vi "ni579x Amplitude Data Interpolator.vi"(8 "Error In":errorcluster, 9 "attenuation index":dbl, 10 "frequency [Hz]":dbl format="%#_6p", 11 "characterization data":T1 {"Frequencies [Hz]" format="%#_6p"}) -> (0 "Error Out":errorcluster, 1 "attenuator values [dB]":dbl[](array[numeric]), 2 "amplitude data":dbl)   [LabVIEW 2013]
uses:
  <instrlib>/ni579x/Config/v1/Shared/Types/ni579x Characterization Data.ctl
  <instrlib>/ni579x/Config/v1/Shared/Types/ni579x IQ Imbalance.ctl
  <instrlib>/ni579x/Config/v1/Shared/Types/ni579x Gain to Attenuation Mapping.ctl
  <vilib>/gmath/interp.llb/Interpolate 2D (1d xi,yi).vi
  <vilib>/gmath/NI_Gmath.lvlib
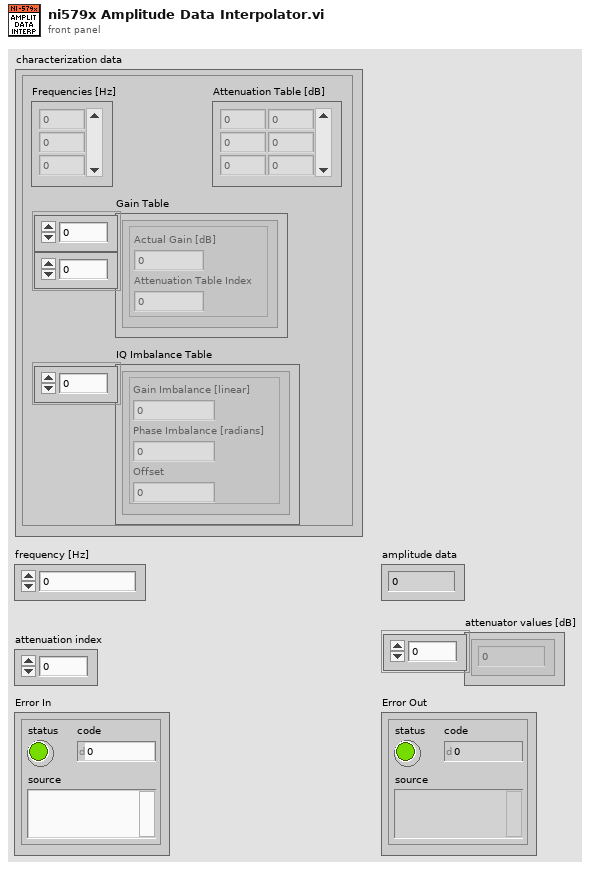
[diagram p1: front panel]
types:
  T1 = typedef "ni579x Characterization Data.ctl" = cluster{"Attenuation Table [dB]":dbl[][], "Frequencies [Hz]":dbl[], "IQ Imbalance Table":T2[], "Gain Table":T3[][]}
  T2 = typedef "ni579x IQ Imbalance.ctl" = cluster{"Gain Imbalance [linear]":dbl, "Phase Imbalance [radians]":dbl, "Offset":cdb}
  T3 = typedef "ni579x Gain to Attenuation Mapping.ctl" = cluster{"Actual Gain [dB]":dbl, "Attenuation Table Index":i32}
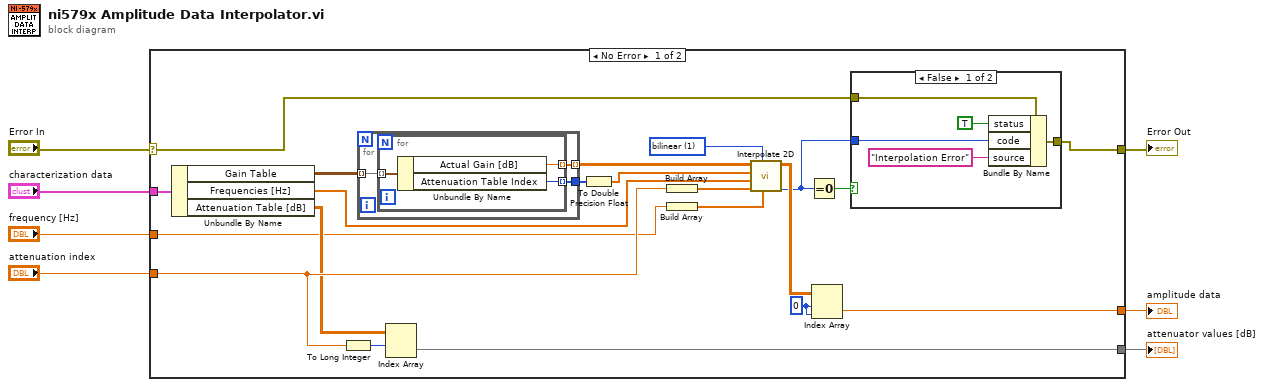
[diagram p0: block diagram]
diagram:
  n1 = case shown="No Error" "Error In" {
    selector: "Error In" -> [w15 w41]
    tunnel: [w11 w41] -> w1
    tunnel: [w28 _] -> w4
    tunnel: "attenuation index" -> [w27 _]
    tunnel: "characterization data" -> [w23 _]
    tunnel: "frequency [Hz]" -> [w8 _]
    tunnel: [w14 _] -> w5
    frame No Error {
      w18 = 1 items=["nearest", "bilinear", "bicubic", "bicubic spline"] ("method")
      w19 = 0 ("index (row)")
      n2 = Unbundle By Name(w23) -> ("Gain Table"=w25:T3[][], "Frequencies [Hz]"=w12:dbl[], "Attenuation Table [dB]"=w13:dbl[][])
      n3 = To Long Integer(number=w27) -> (32bit integer=w26:i32)
      n4 = for {
        tunnel: w25 -> [w37] mode=indexing
        tunnel: [w36] -> w21 mode=indexing
        tunnel: [w35] -> w24
        n5 = for {
          tunnel: w37 -> [w40] mode=indexing
          tunnel: [w39] -> w36 mode=indexing
          tunnel: [w38] -> w35 mode=indexing
          n6 = Unbundle By Name(w40) -> ("Actual Gain [dB]"=w39:dbl, "Attenuation Table Index"=w38:i32)
        }
      }
      n7 = Index Array(array=w13, index (row)=w26) -> (element=w14:dbl[])  [unwired: 1 in]
      n8 = To Double Precision Float(number=w24) -> (double precision float=w22:dbl[])
      n9 = Build Array(w27) -> (w9:dbl[])
      n10 = Build Array(w8) -> (w10:dbl[])
      n11 = call-poly <vilib>:"Interpolate 2D.vi"("yi"=w10, "method"=w18, "xi"=w9, "Y"=w12, "X"=w22, "Z"=w21) -> ("error"=w16:i32, "zi"=w20:dbl[][])  [unwired: 2 in, 2 out]
      n12 = Equal To 0?(x=w16) -> (x = 0?=w17:bool)
      n13 = Index Array(array=w20, index (row)=w19, index (col)=w19) -> (element=w28:dbl)
      n14 = case shown="False" w17 {
        tunnel: w15 -> [w33 w34]
        tunnel: [w32 w34] -> w11
        tunnel: w16 -> [w31 _]
        frame False {
          n15 = Bundle By Name(cluster=w33, "status"=TRUE, "code"=w31, "source"="Interpolation Error") -> (w32:errorcluster)
        }
        frame True {
        }
      }
    }
    frame Error {
    }
  }
  "attenuator values [dB]" <- w5
  "amplitude data" <- w4
  "Error Out" <- w1
